vi "ImportProject.vi"(8 "error in (no error)":errorcluster, 11 "BrowerController in":refnum<class "BrowerController.lvclass">) -> (0 "error out":errorcluster, 3 "BrowerController out":refnum<class "BrowerController.lvclass">)   [LabVIEW 2015, in "BrowerController.lvclass"]
uses:
  BrowerController.lvclass
  BrowerController.lvclass/BrowerController.ctl
  File IO/Controllers/Messages/LoadProject_Msg/LoadProject_Msg.lvclass/LoadProject_Msg.ctl
  <vilib>/ActorFramework/Message Enqueuer/Message Enqueuer.lvclass/Message Enqueuer.ctl
  <vilib>/ActorFramework/Message Enqueuer/Enqueue.vi
  <vilib>/ActorFramework/Message Priority Queue/Priority Enqueue.vi
  File IO/Controllers/Messages/LoadProject_Msg/LoadProject_Msg.lvclass
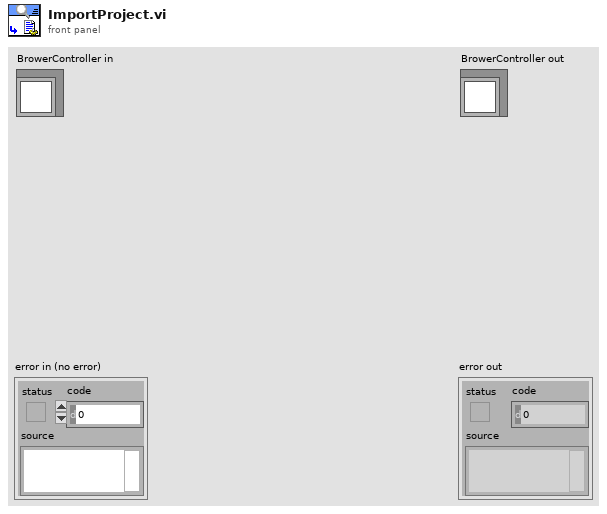
[diagram p1: front panel]
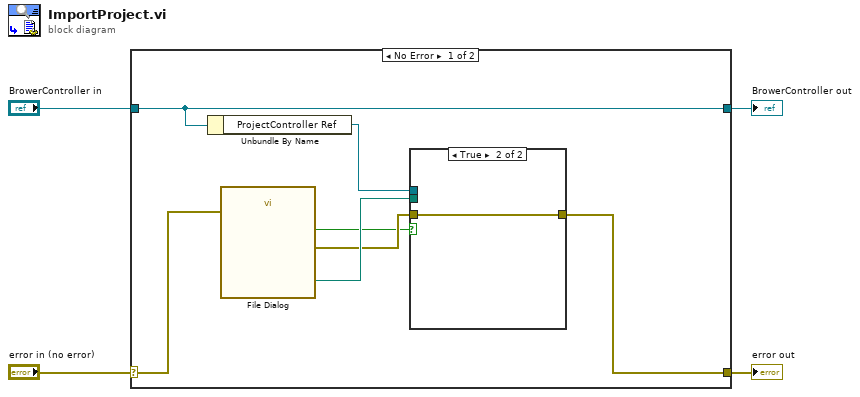
[diagram p0: block diagram]
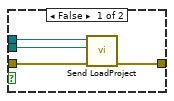
[diagram p2: hidden frame]
diagram:
  n1 = case shown="No Error" "error in (no error)" {
    selector: "error in (no error)" -> [w8 w18]
    tunnel: [w6 w18] -> w3
    tunnel: [w11 w17] -> w1
    tunnel: "BrowerController in" -> [w11 w17]
    frame No Error {
      n2 = Unbundle By Name(w11) -> ("ProjectController Ref"=w10:refnum<class "Message Enqueuer.lvclass">)
      n3 = call "File Dialog"("error in"=w8) -> ("selected path"=w9:path, "cancelled"=w5:bool, "error out"=w7:errorcluster)  [unwired: 11 in, 1 out]
      n4 = case shown="True" w5 {
        tunnel: w10 -> [w15 _]
        tunnel: w9 -> [w14 _]
        tunnel: w7 -> [w13 w16]
        tunnel: [w12 w16] -> w6
        frame False {
          n5 = call "Send LoadProject.vi"("error in (no error)"=w13, "ProjectPath"=w14, "Message Enqueuer"=w15) -> ("error out"=w12:errorcluster)  [unwired: 7 in, 1 out]
        }
        frame True {
        }
      }
    }
    frame Error {
    }
  }
  "error out" <- w3
  "BrowerController out" <- w1
